vi "Scan and Trace(Unfold).vi"() -> ()   [LabVIEW 2020]
uses:
  <vilib>/Utility/error.llb/DialogType.ctl
  Global Parameters.vi
  <vilib>/DAQmx/miscellaneous.llb/DAQmx Fill In Error Info.vi
  <vilib>/DAQmx/configure/timing.llb/DAQmx Timing (Sample Clock).vi
  <vilib>/DAQmx/create/channels.llb/DAQmx Create Channel (CI-Count Edges).vi
  <vilib>/DAQmx/read.llb/DAQmx Read (Counter 1D U32 1Chan NSamp).vi
  <vilib>/Utility/file.llb/Write Delimited Spreadsheet (DBL).vi
  <resource>/objmgr/daqmx.rc
panel:
  in  "Move Wait Time":i32=70
  out "Move Time":u32=103
  in  "milliseconds to wait":u32
  out "Read + Move Time":u32=103
  out "Laser On":bool
  out "Current Position":dbl[](array[numeric])=[100.0, 99.99645996, 110.0]
  in  "stop":bool
  in  "Tab Control":T1(tab)
  in  "Graph path":path=path "I:/scan map test"
  out "Intensity Graph":dbl[][](graph)=[[95300.0, 98850.0, 103700.0, 104550.0, 102500.0, 51500.0, 51850.0, 19000.0, 20650.0, 15000.0, 15300.0, 17150.0, 16250.0, 17200.0, 14950.0, 15050.0, 17650.0, 15350.0, 14300.0, 14550.0, 15700.0], [77600.0, 97750.0, 99400.0, 99250.0, 95500.0, 53250.0, 25650.0, 18800.0, 17350.0, 14250.0, 17250.0, 16050.0, 15600.0, 15200.0, 15250.0, 15700.0, 15150.0, 14650.0, 15600.0, 15700.0, 16550.0], [97000.0, 96100.0, 101550.0, 99100.0, 97250.0, 50150.0, 23650.0, 21050.0, 17550.0, 15950.0, 15300.0, 14700.0, 15200.0, 16950.0, 14500.0, 15450.0, 14550.0, 17050.0, 14550.0, 14900.0, 16600.0], [95600.0, 95800.0, 102500.0, 99350.0, 94900.0, 52700.0, 26600.0, 21250.0, 16250.0, 16150.0, 14800.0, 15550.0, 15800.0, 16350.0, 15400.0, 15850.0, 14500.0, 14750.0, 15550.0, 15750.0, 14900.0], [100050.0, 96100.0, 94400.0, 100500.0, 94450.0, 54350.0, 23850.0, 18950.0, 16100.0, 14850.0, 16700.0, 14950.0, 14250.0, 16700.0, 16100.0, 15700.0, 16450.0, 14650.0, 16950.0, 14000.0, 15800.0], [100300.0, 96050.0, 96850.0, 98000.0, 90700.0, 51250.0, 23450.0, 18050.0, 18300.0, 17300.0, 17050.0, 16300.0, 15950.0, 14850.0, 15500.0, 16450.0, 16200.0, 17200.0, 16450.0, 15300.0, 17100.0], [95650.0, 95650.0, 100700.0, 98700.0, 94500.0, 53950.0, 25250.0, 18850.0, 17150.0, 16050.0, 15050.0, 15450.0, 16050.0, 14600.0, 16500.0, 16350.0, 15500.0, 15450.0, 15300.0, 15150.0, 15650.0], [96700.0, 96200.0, 96650.0, 103650.0, 93400.0, 53300.0, 22500.0, 19050.0, 15850.0, 15350.0, 16550.0, 15200.0, 15250.0, 15400.0, 16550.0, 13950.0, 15150.0, 15600.0, 15150.0, 14500.0, 15900.0], [97500.0, 98050.0, 101500.0, 101650.0, 97000.0, 53700.0, 23400.0, 19450.0, 16700.0, 16850.0, 16450.0, 16250.0, 15900.0, 14600.0, 15700.0, 15400.0, 14900.0, 15950.0, 15450.0, 16050.0, 16100.0], [95400.0, 97550.0, 102050.0, 98600.0, 92100.0, 61200.0, 24550.0, 20500.0, 16000.0, 15350.0, 14450.0, 14150.0, 15750.0, 15950.0, 15750.0, 14800.0, 15000.0, 16150.0, 17250.0, 15350.0, 17400.0], [95750.0, 92950.0, 96100.0, 96550.0, 92550.0, 90100.0, 21900.0, 23000.0, 15000.0, 15550.0, 16000.0, 16000.0, 15400.0, 14150.0, 14350.0, 15950.0, 17250.0, 15750.0, 16100.0, 15300.0, 14400.0]]
  in  "go to crusor":bool caption="X"
  in  "vertical num":u32=20
  in  "horizontal num":u32=10
  in  "horizontal range":dbl=50.0
  in  "horizontal start":dbl=50.0
  in  "vertical range":dbl=200.0
  in  "vertical start":dbl
  in  "Horizontal axis":i8(ring) items=["x", "y", "z", ""]
  in  "Vertical axis":i8(ring)=2 items=["x", "y", "z", ""]
  out "vertical step":dbl=10.0
  out "horizontal step":dbl=5.0
  in  "Stop scan":bool
  out "counts/s":dbl=14400.0 format="%#.10g"
  out "H goal position":dbl[](array[numeric])=[50.0, 55.0, 60.0, 65.0, 70.0, 75.0, 80.0, 85.0, 90.0, 95.0, 100.0]
  out "V goal position":dbl[](array[numeric])=[0.0, 10.0, 20.0, 30.0, 40.0, 50.0, 60.0, 70.0, 80.0, 90.0, 100.0, 110.0, 120.0, 130.0, 140.0, 150.0, 160.0, 170.0, 180.0, 190.0, 200.0]
  out "Loop  indicator":i32=2147483647
  out "Waveform Chart":dbl(graph)=93500.0
  in  "Start moving":bool=TRUE
  in  "Save trace data?":bool
  in  "-0.05 2":bool caption="X"
  in  "Tracing axis":enum16{"x", "y", "z"}(ring)=enum."z"
  in  "-01 2":bool caption="X"
  in  "Wait time(ms)":u32
  in  "+01 2":bool caption="X"
  in  "+0.05 2":bool caption="X"
  in  "-0.01 2":bool caption="X"
  in  "+0.01 2":bool caption="X"
  in  "Exit Tracing":bool
  out "counts rate":dbl=93500.0 format="%#.10g"
  in  "Trace data file path 2":path=path "trace data"
  in  "set trace data save rate(ms)":u32
  in  "Stop Counts":bool
  out "Actual Duty Cycle":dbl=0.5
  out "Actual Frequency":dbl=50.0
  out "Duty Cycle":dbl=0.5 format="%.6f"
  out "Frequency":dbl=50.0 format="%.6f"
  out "Output Terminal":tag="/Dev1/PFI2"
  out "Counter":tag="Dev1/ctr0"
  out "Clock on":bool
  out "ASG连接状态":bool
  out "ASG error":errorcluster
  out "Scanner\n error":errorcluster
  out "Sample Clock Source":tag="/Dev1/PFI2"
  out "Sample Rate":dbl=50.0
  in  "Counter 2":tag="Dev1/ctr1"
  in  "Input Terminal":tag="/Dev1/PFI12"
  in  "Samples":i32=2
  out "Data":u32[](array[numeric])=[293, 581]
  in  "Active Edge":i32(ring)=10280 items=["Rising"=10280, "Falling"=10171]
  in  "Sample Mode":i32(ring)=10178 items=["Finite Samples"=10178, "Continuous Samples"=10123, "Hardware Timed Single Point"=12522]
  in  "start":bool
  in  "Select Process Before Start":enum16{"Goto cursor", "Trace", "Scan"}(ring)=enum."Trace"
  out "Scanning":bool
  out "Tracing":bool
  out "Goto cursor":bool
  # "Only for showing Clock Settings, Please go to Global Parameter to Change the Settings"
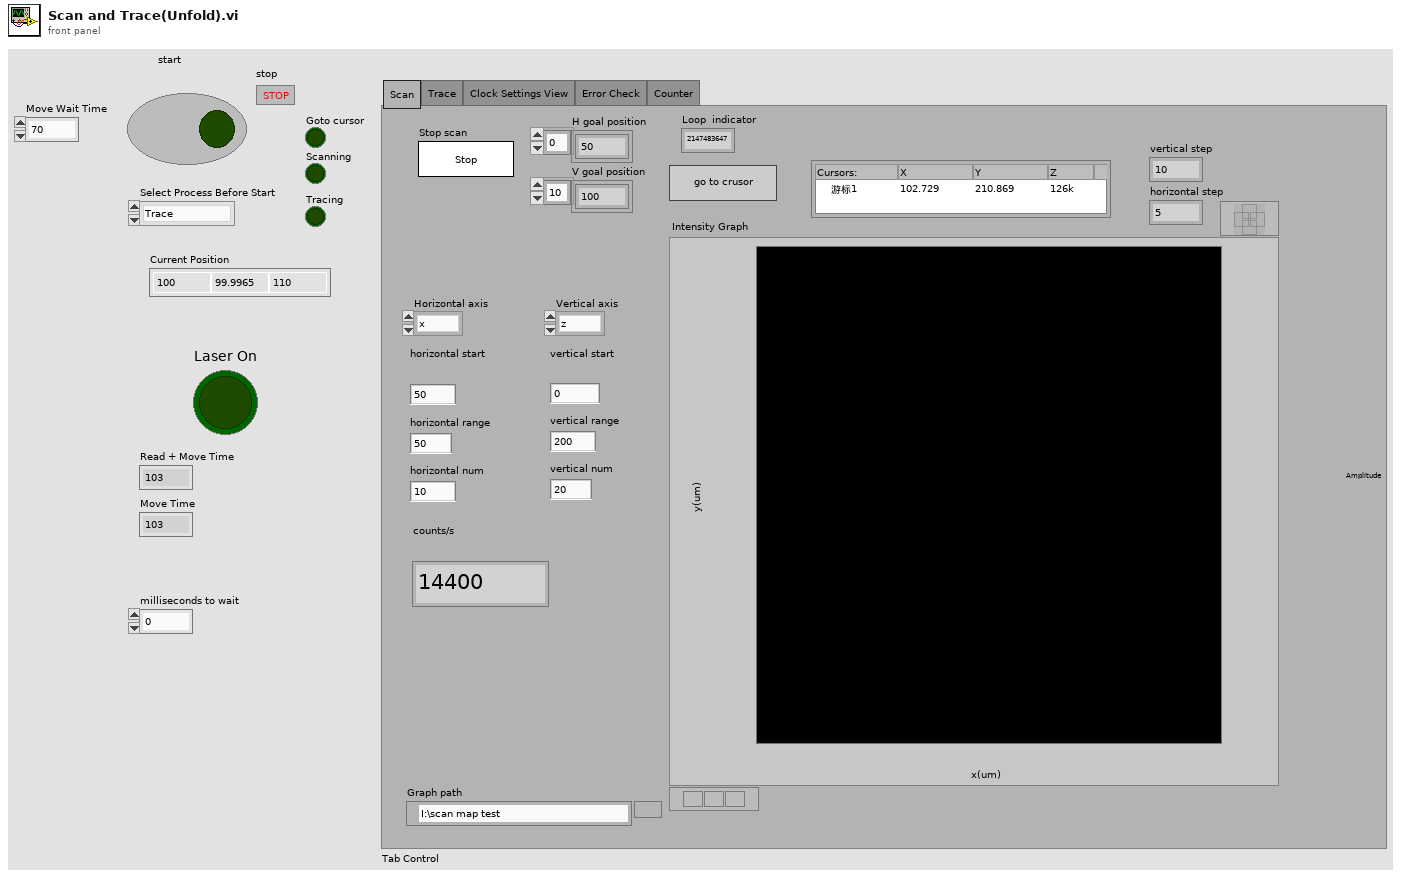
[diagram p1: front panel]
types:
  T1 = enum32{"Scan", "Trace", "Clock Settings View", "Error Check", "Counter"}
  T2 = typedef "DialogType.ctl" = u16
  T3 = typedef "imagedata.ctl" = cluster{"image type":i32, "image depth":i32, "image":u8[], "mask":u8[], "colors":u32[], "Rectangle":cluster{"left":i16, "top":i16, "right":i16, "bottom":i16}}
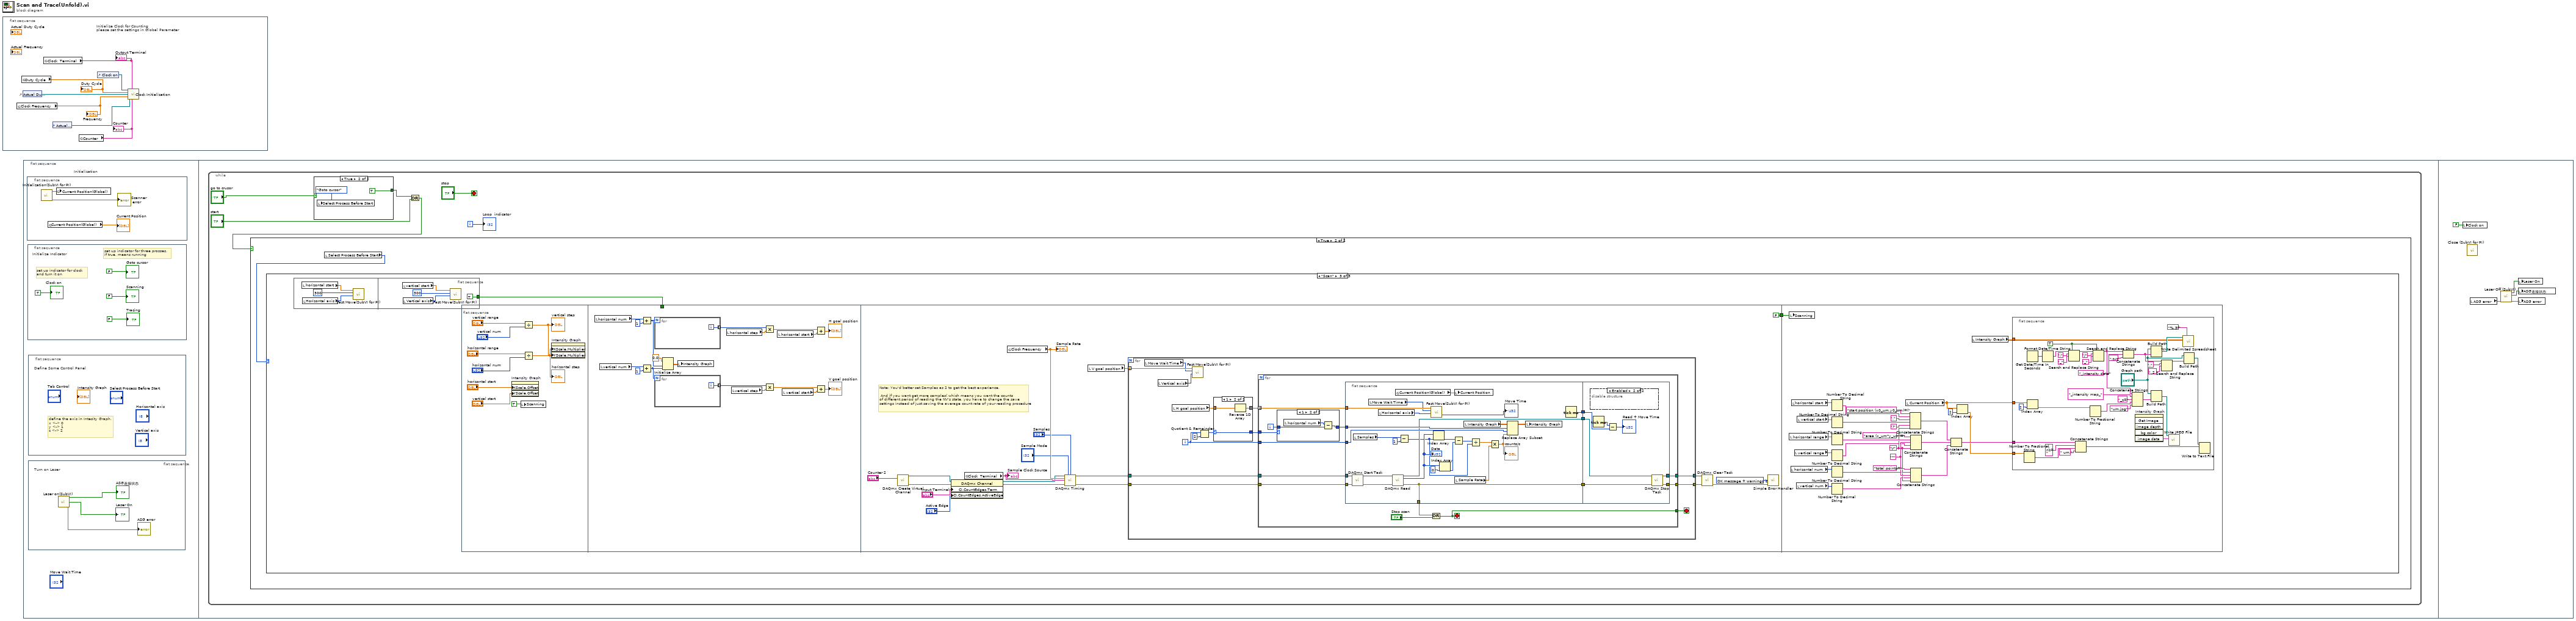
[diagram p0: block diagram]
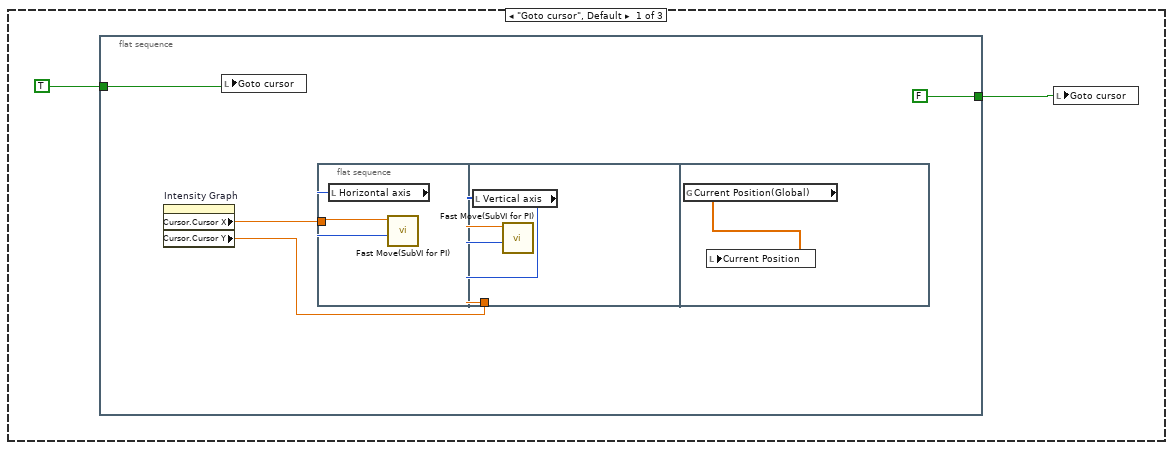
[diagram p3: hidden frame]
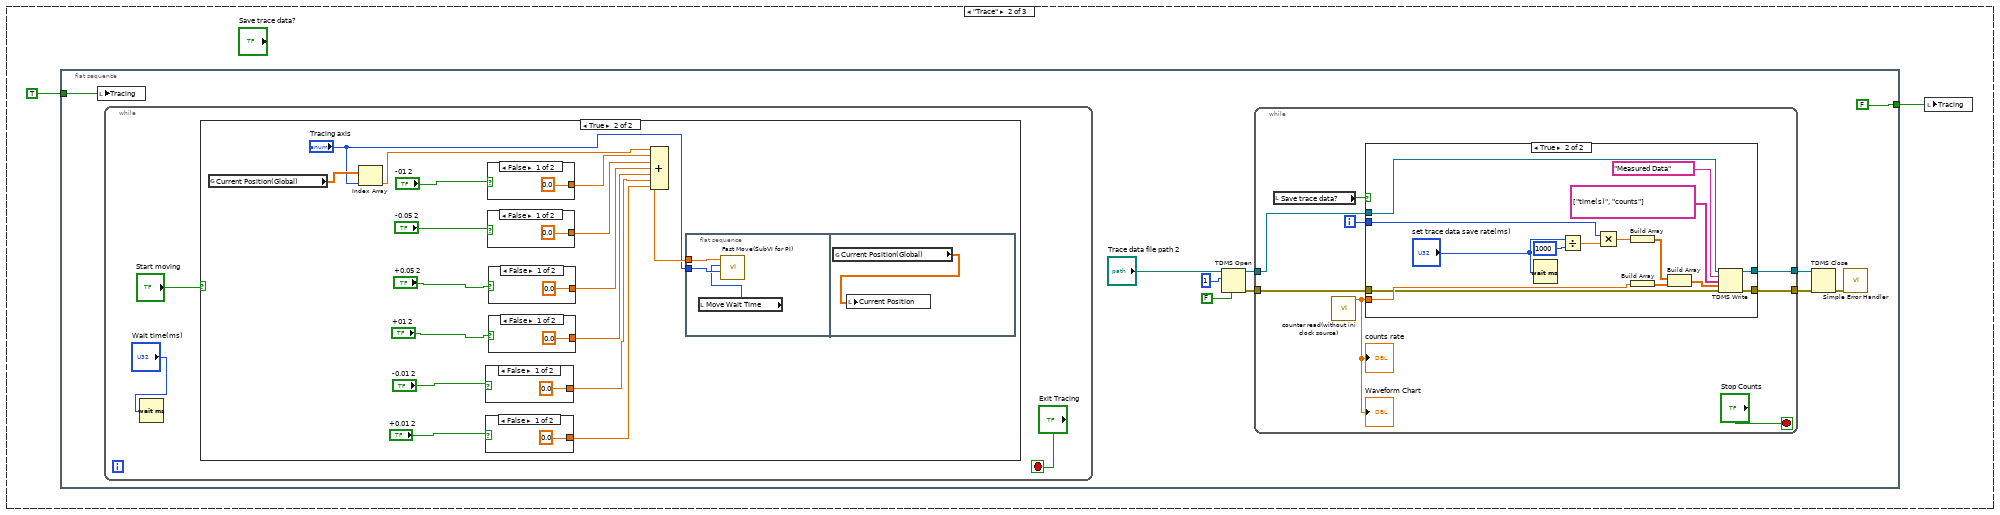
[diagram p4: hidden frame]
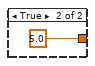
[diagram p7: hidden frame]
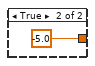
[diagram p8: hidden frame]
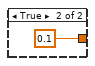
[diagram p9: hidden frame]
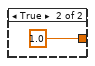
[diagram p10: hidden frame]
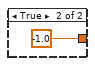
[diagram p11: hidden frame]
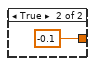
[diagram p12: hidden frame]
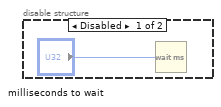
[diagram p14: hidden frame]
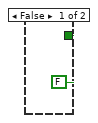
[diagram p16: hidden frame]
diagram:
  n1 = flat-sequence {
    frame #0 {
      # "Initialize Clock for Counting\nplease set the settings in Global Parameter"
      n2 = global read "Global Parameters.vi" "Clock Frequency"() -> (w3:dbl)
      "Frequency" <- w3
      n3 = global read "Global Parameters.vi" "Duty Cycle"() -> (w4:dbl)
      "Duty Cycle" <- w4
      n4 = control-ref of="Actual Duty Cycle"() -> (w1:refnum<vi>)
      n5 = global read "Global Parameters.vi" "Clock  Terminal"() -> (w5:tag)
      "Output Terminal" <- w5
      n6 = control-ref of="Actual Frequency"() -> (w2:refnum<vi>)
      n7 = global read "Global Parameters.vi" "Counter"() -> (w6:tag)
      "Counter" <- w6
      n8 = control-ref of="Clock on"() -> (w7:refnum<vi>)
      n9 = call "Clock Initialization.vi"("Boolean in"=w7, "Output Terminal"=w5, "Duty Cycle"=w4, "Actual Duty Cycle"=w1, "Frequency"=w3, "Actual Frequency"=w2, "Counter"=w6) -> ()  [unwired: 9 in]
    }
  }
  n10 = flat-sequence {
    frame #0 {
      # "Initialization"
      n11 = flat-sequence {
        frame #0 {
          n12 = call "Initialization(SubVI for PI).vi"() -> ("error out"=→"Scanner\n error":errorcluster, "Position"=w16:dbl[])  [unwired: 10 in]
          n13 = global read "Global Parameters.vi" "Current Position(Global)"() -> (→"Current Position":dbl[])
          n14 = global write "Global Parameters.vi" "Current Position(Global)"(w16) -> ()
        }
      }
      n15 = flat-sequence {
        frame #0 {
          # "Initialize Indicator"
          # "set up indicator for clock \nand turn it on"
          # "set up indicator for three prosses,\nif true, means running"
          "Goto cursor" <- FALSE
          "Tracing" <- FALSE
          "Scanning" <- FALSE
          "Clock on" <- TRUE
        }
      }
      n16 = flat-sequence {
        frame #0 {
          # "Define Some Control Panel"
          # "define the axis in Intesity Graph,\nx <-> 0\ny <-> 1\nz <-> 2"
        }
      }
      n17 = flat-sequence {
        frame #0 {
          # "Turn on Laser"
          n18 = call "Laser on(SubVI).vi"() -> ("error out"=→"ASG error":errorcluster, "Laser On"=→"Laser On":bool, "ASG Connection On?"=→"ASG连接状态":bool)  [unwired: 9 in]
        }
      }
    }
    frame #1 {
      n19 = while {
        i -> [w21]
        stop <- "stop" stop-if-true
        n20 = case shown="True" "go to crusor" {
          tunnel: [FALSE TRUE] -> w19
          frame False {
          }
          frame True {
            n21 = local write "Select Process Before Start"(enum16{"Goto cursor", "Trace", "Scan"}."Goto cursor" ("Select Process Before Start")) -> ()
          }
        }
        n22 = Or(x=w19, y="start") -> (x .or. y?=w18:bool)
        n23 = case shown="True" w18 {
          frame False {
          }
          frame True {
            n24 = local read "Select Process Before Start"() -> (w24:enum16{"Goto cursor", "Trace", "Scan"})
            n25 = case shown="\"Scan\"" w24 {
              frame "Goto cursor", Default {
                n26 = flat-sequence {
                  tunnel: TRUE -> [w28]
                  tunnel: [FALSE] -> w25
                  frame #0 {
                    n27 = property on="Intensity Graph" class="IntGraph (strict)"() -> ("Cursor.Cursor X"=w30:dbl, "Cursor.Cursor Y"=w29:dbl)  [unwired: 2 in, 2 out]
                    n28 = local write "Goto cursor"(w28) -> ()
                    n29 = flat-sequence {
                      tunnel: w30 -> [w32]
                      tunnel: w29 -> [w34]
                      frame #0 {
                        n30 = local read "Horizontal axis"() -> (w31:i8)
                        n31 = call "Fast Move(SubVI for PI).vi"("Axes"=w31, "Goal Position"=w32) -> ()  [unwired: 4 in, 2 out]
                      }
                      frame #1 {
                        n32 = local read "Vertical axis"() -> (w33:i8)
                        n33 = call "Fast Move(SubVI for PI).vi"("Axes"=w33, "Goal Position"=w34) -> ()  [unwired: 4 in, 2 out]
                      }
                      frame #2 {
                        n34 = global read "Global Parameters.vi" "Current Position(Global)"() -> (w35:dbl[])
                        n35 = local write "Current Position"(w35) -> ()
                      }
                    }
                  }
                }
                n36 = local write "Goto cursor"(w25) -> ()
              }
              frame "Trace" {
                n37 = flat-sequence {
                  tunnel: [FALSE] -> w37
                  tunnel: TRUE -> [w38]
                  frame #0 {
                    n38 = local write "Tracing"(w38) -> ()
                    n39 = while {
                      stop <- "Exit Tracing" stop-if-true
                      n40 = Wait (ms)(milliseconds to wait="Wait time(ms)") -> ()  [unwired: 1 out]
                      n41 = case shown="True" "Start moving" {
                        frame False {
                        }
                        frame True {
                          n42 = global read "Global Parameters.vi" "Current Position(Global)"() -> (w91:dbl[])
                          n43 = Index Array(array=w91, index="Tracing axis") -> (element=w84:dbl)
                          n44 = case shown="False" "-0.01 2" {
                            tunnel: [0.0 -5.0] -> w86
                            frame False {
                            }
                            frame True {
                            }
                          }
                          n45 = case shown="False" "+0.01 2" {
                            tunnel: [0.0 5.0] -> w85
                            frame False {
                            }
                            frame True {
                            }
                          }
                          n46 = case shown="False" "-01 2" {
                            tunnel: [0.0 -0.1] -> w90
                            frame False {
                            }
                            frame True {
                            }
                          }
                          n47 = case shown="False" "-0.05 2" {
                            tunnel: [0.0 -1.0] -> w89
                            frame False {
                            }
                            frame True {
                            }
                          }
                          n48 = case shown="False" "+0.05 2" {
                            tunnel: [0.0 1.0] -> w88
                            frame False {
                            }
                            frame True {
                            }
                          }
                          n49 = case shown="False" "+01 2" {
                            tunnel: [0.0 0.1] -> w87
                            frame False {
                            }
                            frame True {
                            }
                          }
                          n50 = Compound Arithmetic op=ADD(w84, w90, w89, w88, w87, w86, w85) -> (w77:dbl)
                          n51 = flat-sequence {
                            tunnel: w77 -> [w106]
                            tunnel: "Tracing axis" -> [w105]
                            frame #0 {
                              n52 = local read "Move Wait Time"() -> (w104:i32)
                              n53 = call "Fast Move(SubVI for PI).vi"("Axes"=w105, "Milliseconds to wait"=w104, "Goal Position"=w106) -> ()  [unwired: 3 in, 2 out]
                            }
                            frame #1 {
                              n54 = global read "Global Parameters.vi" "Current Position(Global)"() -> (w107:dbl[])
                              n55 = local write "Current Position"(w107) -> ()
                            }
                          }
                        }
                      }
                    }
                    n56 = TDMS Open(6:FALSE ("disable buffering (T)"), 10:1, 11:"Trace data file path 2") -> (0:w45:errorcluster, 3:w44:refnum<k34>)  [unwired: 4 in]
                    n57 = while {
                      tunnel: w45 -> [w54]
                      tunnel: w44 -> [w53]
                      tunnel: [w50] -> w42
                      tunnel: [w49] -> w41
                      i -> [w55]
                      stop <- "Stop Counts" stop-if-true
                      n58 = local read "Save trace data?"() -> (w51:bool)
                      n59 = call "counter read(without ini clock source).vi"() -> ("counter rate"=w52:dbl)  [unwired: 11 in]
                      "counts rate" <- w52
                      "Waveform Chart" <- w52
                      n60 = case shown="True" w51 {
                        tunnel: w53 -> [w57 w64]
                        tunnel: [w57 w63] -> w50
                        tunnel: w52 -> [_ w62]
                        tunnel: w54 -> [w56 w61]
                        tunnel: [w56 w60] -> w49
                        tunnel: w55 -> [_ w59]
                        frame False {
                        }
                        frame True {
                          n61 = Wait (ms)(milliseconds to wait="set trace data save rate(ms)") -> ()  [unwired: 1 out]
                          n62 = Divide(x="set trace data save rate(ms)", y=u32 1000) -> (x/y=w66:dbl)
                          n63 = Multiply(x=w59, y=w66) -> (x*y=w65:dbl)
                          n64 = Build Array(w65) -> (w70:dbl[])
                          n65 = Build Array(w62) -> (w69:dbl[])
                          n66 = Build Array(w70, w69) -> (w68:dbl[][])
                          n67 = TDMS Write(0:w64, 5:"Measured Data" ("group name"), 7:string[] ["time(s)", "counts"] ("channel names"), 9:w68, 11:w61) -> (4:w63:refnum<k34>, 15:w60:errorcluster)  [unwired: 1 in, 2 out]
                        }
                      }
                    }
                    n68 = TDMS Close(8:w41, 11:w42) -> (0:w43:errorcluster)  [unwired: 1 out]
                    n69 = call <vilib>:"Simple Error Handler.vi"("error in (no error)"=w43) -> ()  [unwired: 1 in, 8 out]
                  }
                }
                n70 = local write "Tracing"(w37) -> ()
              }
              frame "Scan" {
                n71 = flat-sequence {
                  tunnel: [TRUE] -> w108
                  frame #0 {
                    n72 = local read "horizontal start"() -> (w112:dbl)
                    n73 = local read "Horizontal axis"() -> (w111:i8)
                    n74 = call "Fast Move(SubVI for PI).vi"("Axes"=w111, "Milliseconds to wait"=300, "Goal Position"=w112) -> ()  [unwired: 3 in, 2 out]
                  }
                  frame #1 {
                    n75 = local read "vertical start"() -> (w116:dbl)
                    n76 = local read "Vertical axis"() -> (w115:i8)
                    n77 = call "Fast Move(SubVI for PI).vi"("Axes"=w115, "Milliseconds to wait"=300, "Goal Position"=w116) -> ()  [unwired: 3 in, 2 out]
                  }
                }
                n78 = flat-sequence {
                  tunnel: w108 -> [_]
                  tunnel: [FALSE] -> w109
                  tunnel: w109 -> [w265]
                  frame #0 {
                    n79 = property on="Intensity Graph" class="IntGraph (strict)"("XScale.Offset"="horizontal start", "YScale.Offset"="vertical start") -> ()  [unwired: 2 in, 2 out]
                    n80 = local write "Scanning"(TRUE) -> ()
                    n81 = Divide(x="vertical range", y="vertical num") -> (x/y=w117:dbl)
                    "vertical step" <- w117
                    n82 = Divide(x="horizontal range", y="horizontal num") -> (x/y=w118:dbl)
                    "horizontal step" <- w118
                    n83 = property on="Intensity Graph" class="IntGraph (strict)"("XScale.Multiplier"=w118, "YScale.Multiplier"=w117) -> ()  [unwired: 2 in, 2 out]
                  }
                  frame #1 {
                    n84 = local read "horizontal num"() -> (w128:u32)
                    n85 = local read "vertical num"() -> (w131:u32)
                    n86 = Add(x=w128, y=1) -> (x+y=w127:u32)
                    n87 = Add(x=w131, y=1) -> (x+y=w126:u32)
                    n88 = for {
                      N: w127 -> [_]
                      tunnel: [w145] -> w143 mode=indexing
                      i -> [w145]
                    }
                    n89 = for {
                      N: w126 -> [_]
                      tunnel: [w144] -> w138 mode=indexing
                      i -> [w144]
                    }
                    n90 = Initialize Array(0.0, w127, w126) -> (w132:dbl[][])
                    n91 = local write "Intensity Graph"(w132) -> ()
                    n92 = local read "horizontal step"() -> (w142:dbl)
                    n93 = local read "vertical step"() -> (w137:dbl)
                    n94 = Multiply(x=w143, y=w142) -> (x*y=w141:dbl[])
                    n95 = Multiply(x=w138, y=w137) -> (x*y=w136:dbl[])
                    n96 = local read "horizontal start"() -> (w140:dbl)
                    n97 = local read "vertical start"() -> (w135:dbl)
                    n98 = Add(x=w141, y=w140) -> (x+y=→"H goal position":dbl[])
                    n99 = Add(x=w136, y=w135) -> (x+y=→"V goal position":dbl[])
                  }
                  frame #2 {
                    w161 = T2 3 items=["no dialog", "OK message", "continue or stop message", "OK message + warnings", "continue/stop + warnings"] ("type of dialog (OK msg:1)")
                    # "Note: You'd better set Samples as 2 to get the best experience,\n\n And if you want get more samples( which means you want the counts \nof different period of reading the NV's state, you have to change the save \nsettings instead of just saving the average count rate of your reading procedure"
                    n100 = call-poly <vilib>:"DAQmx Create Virtual Channel.vi"("counter"="Counter 2") -> ("task out"=w157:refnum<k21>, "error out"=w156:errorcluster)  [unwired: 13 in]
                    n101 = property class="DAQmx Channel"(reference=w157, error in=w156, "CI.CountEdges.Term"="Input Terminal", "CI.CountEdges.ActiveEdge"="Active Edge") -> (reference out=w149:refnum<k21>, error out=w148:errorcluster)
                    n102 = global read "Global Parameters.vi" "Clock  Terminal"() -> (w154:tag)
                    "Sample Clock Source" <- w154
                    n103 = global read "Global Parameters.vi" "Clock Frequency"() -> (w155:dbl)
                    "Sample Rate" <- w155
                    n104 = call-poly <vilib>:"DAQmx Timing.vi"("task/channels in"=w149, "sample mode"="Sample Mode", "samples per channel"="Samples", "rate"=w155, "source"=w154, "error in"=w148) -> ("task out"=w147:refnum<k21>, "error out"=w146:errorcluster)  [unwired: 8 in]
                    n105 = local read "V goal position"() -> (w164:dbl[])
                    n106 = for {
                      tunnel: w164 -> [w172] mode=indexing
                      tunnel: [w167] -> w153
                      tunnel: [w166] -> w152
                      tunnel: w147 -> [w169]
                      tunnel: w146 -> [w168]
                      i -> [w173]
                      stop <- w170 stop-if-true
                      n107 = local read "Move Wait Time"() -> (w165:i32)
                      n108 = local read "Vertical axis"() -> (w171:i8)
                      n109 = local read "H goal position"() -> (w177:dbl[])
                      n110 = call "Fast Move(SubVI for PI).vi"("Axes"=w171, "Milliseconds to wait"=w165, "Goal Position"=w172) -> ()  [unwired: 3 in, 2 out]
                      n111 = Quotient & Remainder(x=w173, y=2) -> (x-y*floor(x/y)=w176:i32)  [unwired: 1 out]
                      n112 = case shown="1" w176 {
                        selector: w176 -> [w233 w235]
                        tunnel: w177 -> [w234 w237]
                        tunnel: [w234 w236] -> w175
                        tunnel: [w233 w235] -> w174
                        frame 0, Default {
                        }
                        frame 1 {
                          n113 = Reverse 1D Array(array=w237) -> (reversed array=w236:dbl[])
                        }
                      }
                      n114 = for {
                        tunnel: w175 -> [w193] mode=indexing
                        tunnel: w174 -> [w192]
                        tunnel: w173 -> [w189]
                        tunnel: [w186] -> w170
                        tunnel: w169 -> [w185]
                        tunnel: w168 -> [w184]
                        tunnel: [w181] -> w167
                        tunnel: [w180] -> w166
                        i -> [w191]
                        stop <- w186 stop-if-true
                        n115 = case shown="1" w192 {
                          tunnel: w191 -> [w194 w196]
                          tunnel: [w194 w195] -> w190
                          frame 0, Default {
                          }
                          frame 1 {
                            n116 = local read "horizontal num"() -> (w197:u32)
                            n117 = Subtract(x=w197, y=w196) -> (x-y=w195:u32)
                          }
                        }
                        n118 = flat-sequence {
                          tunnel: [w215] -> w188
                          tunnel: [w216] -> w183
                          tunnel: [w215] -> w182
                          tunnel: [w202] -> w179
                          tunnel: w184 -> [w217]
                          tunnel: w185 -> [w218]
                          tunnel: w189 -> [w222]
                          tunnel: w193 -> [w201]
                          tunnel: w190 -> [w223]
                          tunnel: w183 -> [w230]
                          tunnel: w182 -> [w229]
                          tunnel: [w228] -> w181
                          tunnel: [w227] -> w180
                          tunnel: w179 -> [w226]
                          frame #0 {
                            n119 = call <vilib>:"DAQmx Start Task.vi"("task/channels in"=w218, "error in"=w217) -> ("task out"=w204:refnum<k21>, "error out"=w203:errorcluster)  [unwired: 12 in]
                            n120 = local read "Samples"() -> (w209:i32)
                            n121 = local read "Move Wait Time"() -> (w198:i32)
                            n122 = local read "Horizontal axis"() -> (w200:i8)
                            n123 = call-poly <vilib>:"DAQmx Read.vi"("task/channels in"=w204, "error in"=w203) -> ("task out"=w216:refnum<k21>, "data"=w208:u32[], "error out"=w215:errorcluster)  [unwired: 11 in]
                            "Data" <- w208
                            n124 = global read "Global Parameters.vi" "Current Position(Global)"() -> (w220:dbl[])
                            n125 = Subtract(x=w209, y=1) -> (x-y=w205:i32)
                            n126 = call "Fast Move(SubVI for PI).vi"("Axes"=w200, "Milliseconds to wait"=w198, "Goal Position"=w201) -> ("Time of move"=→"Move Time":u32)  [unwired: 3 in, 1 out]
                            n127 = Index Array(array=w208, index=w205) -> (element=w211:u32)
                            n128 = Index Array(array=w208, index=0) -> (element=w212:u32)
                            n129 = Subtract(x=w211, y=w212) -> (x-y=w210:u32)
                            n130 = local write "Current Position"(w220) -> ()
                            n131 = local read "Sample Rate"() -> (w206:dbl)
                            n132 = local read "Intensity Graph"() -> (w224:dbl[][])
                            n133 = Divide(x=w210, y=w205) -> (x/y=w207:dbl)
                            n134 = Multiply(x=w207, y=w206) -> (x*y=w219:dbl)
                            "counts/s" <- w219
                            n135 = Replace Array Subset(array=w224, new element=w219, index (row)=w223, index (col)=w222) -> (w221:dbl[][])
                            n136 = local write "Intensity Graph"(w221) -> ()
                            n137 = Tick Count (ms)() -> (millisecond timer value=w202:u32)
                          }
                          frame #1 {
                            n138 = disable-structure shown="Enabled" {
                              frame Disabled {
                                n139 = Wait (ms)(milliseconds to wait="milliseconds to wait") -> ()  [unwired: 1 out]
                              }
                              frame Enabled {
                              }
                            }
                            n140 = Tick Count (ms)() -> (millisecond timer value=w225:u32)
                            n141 = Subtract(x=w225, y=w226) -> (x-y=→"Read + Move Time":u32)
                            n142 = call <vilib>:"DAQmx Stop Task.vi"("task/channels in"=w230, "error in"=w229) -> ("task out"=w228:refnum<k21>, "error out"=w227:errorcluster)  [unwired: 12 in]
                          }
                        }
                        n143 = Or(x=w188, y="Stop scan") -> (x .or. y?=w186:bool)
                      }
                    }
                    n144 = call <vilib>:"DAQmx Clear Task.vi"("task in"=w153, "error in"=w152) -> ("error out"=w162:errorcluster)  [unwired: 13 in]
                    n145 = call <vilib>:"Simple Error Handler.vi"("type of dialog (OK msg:1)"=w161, "error in (no error)"=w162) -> ()  [unwired: 3 in, 5 out]
                  }
                  frame #3 {
                    w254 = "\r"
                    w256 = "*" ("string")
                    n146 = local write "Scanning"(w265) -> ()
                    n147 = local read "horizontal range"() -> (w243:dbl)
                    n148 = local read "horizontal num"() -> (w249:u32)
                    n149 = local read "horizontal start"() -> (w246:dbl)
                    n150 = local read "vertical range"() -> (w242:dbl)
                    n151 = local read "vertical num"() -> (w248:u32)
                    n152 = local read "vertical start"() -> (w245:dbl)
                    n153 = Number To Decimal String(number=w246) -> (decimal integer string=w263:string)  [unwired: 1 out]
                    n154 = Number To Decimal String(number=w245) -> (decimal integer string=w261:string)  [unwired: 1 out]
                    n155 = Number To Decimal String(number=w243) -> (decimal integer string=w258:string)  [unwired: 1 out]
                    n156 = Number To Decimal String(number=w242) -> (decimal integer string=w244:string)  [unwired: 1 out]
                    n157 = Number To Decimal String(number=w249) -> (decimal integer string=w255:string)  [unwired: 1 out]
                    n158 = Number To Decimal String(number=w248) -> (decimal integer string=w247:string)  [unwired: 1 out]
                    n159 = local read "Current Position"() -> (w238:dbl[])
                    n160 = Concatenate Strings("start position (x0_um,y0_um)=(" ("string"), w263, "," ("string"), w261, ")" ("string"), w254) -> (w253:string)
                    n161 = Concatenate Strings("area (x_um*y_um)=" ("string"), w258, w256, w244, w254) -> (w252:string)
                    n162 = Concatenate Strings("total points=" ("string"), w255, w256, w247, w254) -> (w251:string)
                    n163 = Concatenate Strings(w253, w252, w251) -> (w250:string)
                    n164 = Index Array(array=w238, index=2) -> (element=w240:dbl)
                    n165 = local read "Intensity Graph"() -> (w239:dbl[][])
                    n166 = flat-sequence {
                      tunnel: w239 -> [w268]
                      tunnel: w250 -> [w281]
                      tunnel: w240 -> [w279]
                      tunnel: w238 -> [w274]
                      frame #0 {
                        w271 = TRUE ("replace all? (F)")
                        n167 = Number To Fractional String(number=w279) -> (F-format string=w278:string)  [unwired: 3 in]
                        n168 = Get Date/Time In Seconds() -> (seconds since 1Jan1904=w301:timestamp)
                        n169 = Index Array(array=w274, index=2 ("索引")) -> (element=w272:dbl)
                        n170 = Format Date/Time String(seconds (now)=w301) -> (date/time string=w295:string)  [unwired: 2 out]
                        n171 = Search and Replace String(replace all?=w271, input string=w295, search string=":", replace string="_" ("replace string (\"\")")) -> (result string=w298:string)  [unwired: 1 in, 6 out]
                        n172 = Concatenate Strings(w281, "\nz=" ("字符串"), w278, " um." ("字符串")) -> (w280:string)
                        n173 = Number To Fractional String(number=w272) -> (F-format string=w275:string)  [unwired: 3 in]
                        n174 = Search and Replace String(replace all?=w271, input string=w298, search string="/", replace string="_" ("replace string (\"\")")) -> (result string=w286:string)  [unwired: 1 in, 6 out]
                        n175 = Concatenate Strings(w286, "_intensity date" ("string"), ".txt" ("string")) -> (w291:string)
                        n176 = Concatenate Strings(w286, "_intensity map_" ("string"), "_z=" ("字符串"), w275, "um.jpg" ("string")) -> (w294:string)
                        n177 = invoke on="Intensity Graph" class="IntGraph (strict)" method="Get Image"() -> ("image data"=w267:T3)  [unwired: 6 in, 5 out]
                        n178 = Build Path(base path="Graph path", name or relative path=w291) -> (appended path=w269:path)
                        n179 = Build Path(base path="Graph path", name or relative path=w294) -> (appended path=w293:path)
                        n180 = Search and Replace String(input string=w291, search string="." ("substring (\"\")"), replace string="_2." ("replace string (\"\")")) -> (result string=w288:string)  [unwired: 1 in, 7 out]
                        n181 = call <vilib>:"Write JPEG File.vi"("image data"=w267, "path to JPEG file"=w293) -> ()  [unwired: 1 in, 9 out]
                        n182 = call-poly <vilib>:"Write Delimited Spreadsheet.vi"("file path (dialog if empty)"=w269, "format (%.3f)"="%.3f", "2D data"=w268) -> ()  [unwired: 11 in, 2 out]
                        n183 = Build Path(base path="Graph path", name or relative path=w288) -> (appended path=w287:path)
                        n184 = Write to Text File(file (use dialog)=w287, text=w280) -> ()  [unwired: 1 in, 4 out]
                      }
                    }
                  }
                }
              }
            }
          }
        }
        "Loop  indicator" <- w21
      }
    }
    frame #2 {
      n185 = local write "Clock on"(FALSE) -> ()
      n186 = call "Close (SubVI for PI).vi"() -> ()  [unwired: 12 in]
      n187 = local read "ASG error"() -> (w305:errorcluster)
      n188 = call "Laser Off (SubVI).vi"("error in (no error)"=w305) -> ("error out"=w306:errorcluster, "ASG Connection on"=w307:bool, "Laser On"=w308:bool)  [unwired: 8 in]
      n189 = local write "Laser On"(w308) -> ()
      n190 = local write "ASG连接状态"(w307) -> ()
      n191 = local write "ASG error"(w306) -> ()
    }
  }
